vi "S7COMM - Format Write Request.vi"(4 "Bit Offset":u8, 6 "Data":u32[](array[numeric]), 7 "Variable Type":T3=enum."BIT", 8 "Data Block #":u16, 9 "Start Address":T1, 10 "Memory Area":T2 items=["P Area"=128, "I Area"=129, "O Area"=130, "M Area"=131, "DB Area"=132, "Counter"=40, "Timer"=41], 11 "S7":refnum<class "S7NetCom.lvclass">) -> (2 "S7 PDU Data":T4 format="0x%02x", 3 "S7 out":refnum<class "S7NetCom.lvclass">)   [LabVIEW 2014, in "S7NetCom.lvclass"]
doc: "____\nCopyright (c) 2019 Hampel Software Engineering (HSE), released under BSD license. More info can be found on https://dokuwiki.hampel-soft.com/code/hse/s7netcom. Original code published by Marc Christenson, Sisu Devices."
uses:
  S7NetCom.lvclass
  Controls/S7NetCom_HexByteArray.ctl
  Controls/S7NetCom_HexByte.ctl
  Controls/S7_Variable_Type.ctl
  Controls/S7_Memory_Area.ctl
  Controls/S7_Start_Address.ctl
  S7COMM - Function Codes--ring.ctl
  S7NetCom.lvclass/S7NetCom.ctl
  S7COMM - Get Size Factor from Transport Data Type.vi
  S7COMM - Create JOB Message Header.vi
  S7COMM - Header - Protocol ID--constant.vi
panel:
  # "More info on https://dokuwiki.hampel-soft.com/code/hse/s7netcom\n\nCopyright (c) 2019, HAMPEL SOFTWARE ENGINEERING (HSE)\nOriginal code developed by Marc Christenson, Sisu Devices\nAll rights reserved.\n\nRedistribution and use in source and binary forms, with or without\nmodification, are permitted provided that the following conditions are met:\n\n1. Redistributions of source code must retain the above copyright\n   notice, this list of conditions and the following disclaimer.\n\n2. Redistributions in binary form must reproduce the above copyright\n   notice, this list of conditions and the following disclaimer in the\n   documentation and/or other materials provided with the distribution.\n\n3. All advertising materials mentioning features or use of this software\n   must display the following acknowledgement:\n   This product includes software developed by HAMPEL SOFTWARE ENGINEERING.\n\n4. Neither the name of HAMPEL SOFTWARE ENGINEERING nor the\n   names of its contributors may be used to endorse or promote products\n   derived from this software without specific prior written permission.\n\nTHIS SOFTWARE IS PROVIDED BY HAMPEL SOFTWARE ENGINEERING ''AS IS'' AND ANY\nEXPRESS OR IMPLIED WARRANTIES, INCLUDING, BUT NOT LIMITED TO, THE IMPLIED\nWARRANTIES OF MERCHANTABILITY AND FITNESS FOR A PARTICULAR PURPOSE ARE\nDISCLAIMED. IN NO EVENT SHALL HAMPEL SOFTWARE ENGINEERING BE LIABLE FOR ANY\nDIRECT, INDIRECT, INCIDENTAL, SPECIAL, EXEMPLARY, OR CONSEQUENTIAL DAMAGES\n(INCLUDING, BUT NOT LIMITED TO, PROCUREMENT OF SUBSTITUTE GOODS OR SERVICES;\nLOSS OF USE, DATA, OR PROFITS; OR BUSINESS INTERRUPTION) HOWEVER CAUSED AND\nON ANY THEORY OF LIABILITY, WHETHER IN CONTRACT, STRICT LIABILITY, OR TORT\n(INCLUDING NEGLIGENCE OR OTHERWISE) ARISING IN ANY WAY OUT OF THE USE OF THIS\nSOFTWARE, EVEN IF ADVISED OF THE POSSIBILITY OF SUCH DAMAGE."
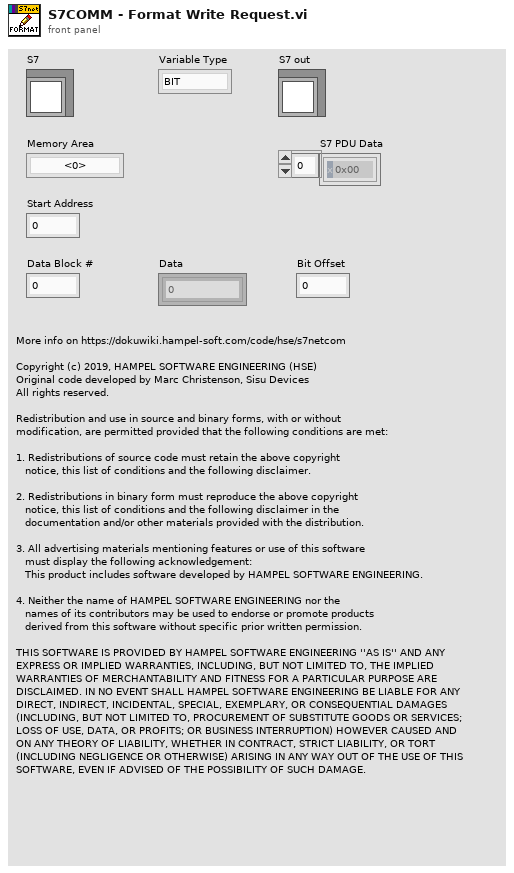
[diagram p1: front panel]
types:
  T1 = typedef "S7NetCom.lvclass/S7_Start_Address.ctl" = u16
  T2 = typedef "S7NetCom.lvclass/S7_Memory_Area.ctl" = u8
  T3 = typedef "S7NetCom.lvclass/S7_Variable_Type.ctl" = enum8{"---", "BIT", "BYTE", "CHAR", "WORD", "INT", "DWORD", "DINT", "REAL"}
  T4 = typedef "S7NetCom.lvclass/S7NetCom_HexByteArray.ctl" = T5[]
  T5 = typedef "S7NetCom.lvclass/S7NetCom_HexByte.ctl" = u8
  T6 = typedef "S7NetCom.lvclass/S7COMM - Function Codes--ring.ctl" = u8
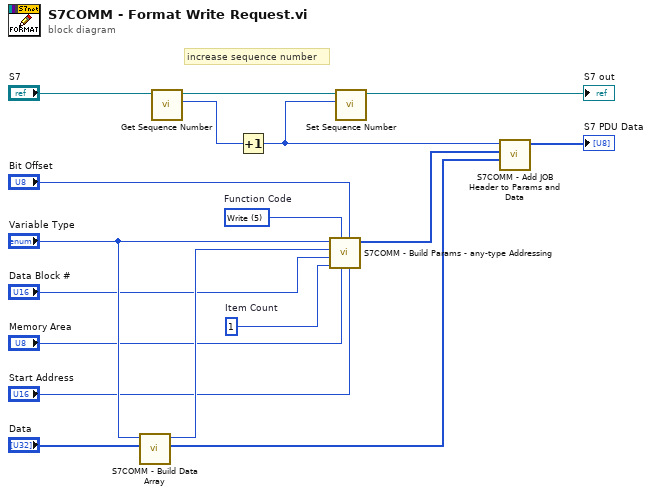
[diagram p0: block diagram]
diagram:
  w2 = u8 1  # Item Count
  w8 = T6 5 items=["Read"=4, "Write"=5]  # Function Code
  # "increase sequence number"
  n1 = call "S7COMM - Build Data Array.vi"("Data"="Data", "Variable Type"="Variable Type") -> ("S7 Data (Byte Array)"=w9:T4, "Data Length"=w6:u16)  [unwired: 8 in]
  n2 = call "Get Sequence Number.vi"("S7NetCom in"="S7") -> ("Sequence No."=w13:u16, "S7NetCom out"=w15:refnum<class "S7NetCom.lvclass">)  [unwired: 9 in]
  n3 = Increment(x=w13) -> (x+1=w11:u16)
  n4 = call "S7COMM - Build Params - any-type Addressing.vi"("Start Address"="Start Address", "Bit Offset"="Bit Offset", "S7_Memory_Area"="Memory Area", "S7_Function_Code"=w8, "Item Count"=w2, "DB Number"="Data Block #", "Count"=w6, "S7_Variable_Type"="Variable Type") -> ("S7 Params Byte Array"=w10:T4)  [unwired: 3 in]
  n5 = call "Set Sequence Number.vi"("Sequence No."=w11, "S7NetCom in"=w15) -> ("S7NetCom out"=→"S7 out":refnum<class "S7NetCom.lvclass">)  [unwired: 9 in]
  n6 = call "S7COMM - Add JOB Header to Params and Data.vi"("S7 Data"=w9, "S7 Parameters"=w10, "Sequence Number"=w11) -> ("S7 PDU"=→"S7 PDU Data":T4)  [unwired: 8 in]
